vi "run.vi"(8 "error in (no error)":errorcluster, 11 "ScanModeMG090624Camera in":refnum<class "ImagingModeMG090624Camera.lvclass">) -> (0 "error out":errorcluster, 3 "ScanModeMG090624Camera out":refnum<class "ImagingModeMG090624Camera.lvclass">)   [LabVIEW 2010, in "ImagingModeMG090624Camera.lvclass"]
uses:
  ImagingModeMG090624Camera.lvclass
  common/xcontrols/XSettings/XSettings/XSettings.xctl
  common/classes/GenericComponent/GenericComponent/GenericComponent.lvclass
  main/labview_source/controls/undock_button.ctl
  ImagingModeMG090624Camera.lvclass/ImagingModeMG090624Camera.ctl
  ImagingModeDL091001Scaffold/ImagingModeDL091001Scaffold/ImagingModeDL091001Scaffold.lvclass
  ImagingModeDL091001Scaffold/ImagingModeDL091001Scaffold/internal_triggers_enum.ctl
  GenericImagingMode/GenericImagingMode/GenericImagingMode.lvclass
panel:
  in  "button:undock":T1
  in  "Tab Control":enum32{"User", "Debug", "About"}(tab)
  in  "frame rate":dbl[unit]=5.0
  in  "y resolution":i32=512
  in  "x resolution":i32=512 min=1
  in  "duration":dbl[unit]
  in  "number of frames":i32
  in  "current frame":i32
  in  "XSettings":refnum<class "GenericComponent.lvclass">(xcontrol)
  out "terminated?":bool
  out "event loop error":errorcluster
  out "XImage is user-defined?":bool
  # "frame settings"
  # "movie settings"
  # "current values"
  # "ImagingModeMG090624Camera\n\nImplemented by:\nMaurice Göldi and Dominik Langer, University of Zürich, Switzerland"
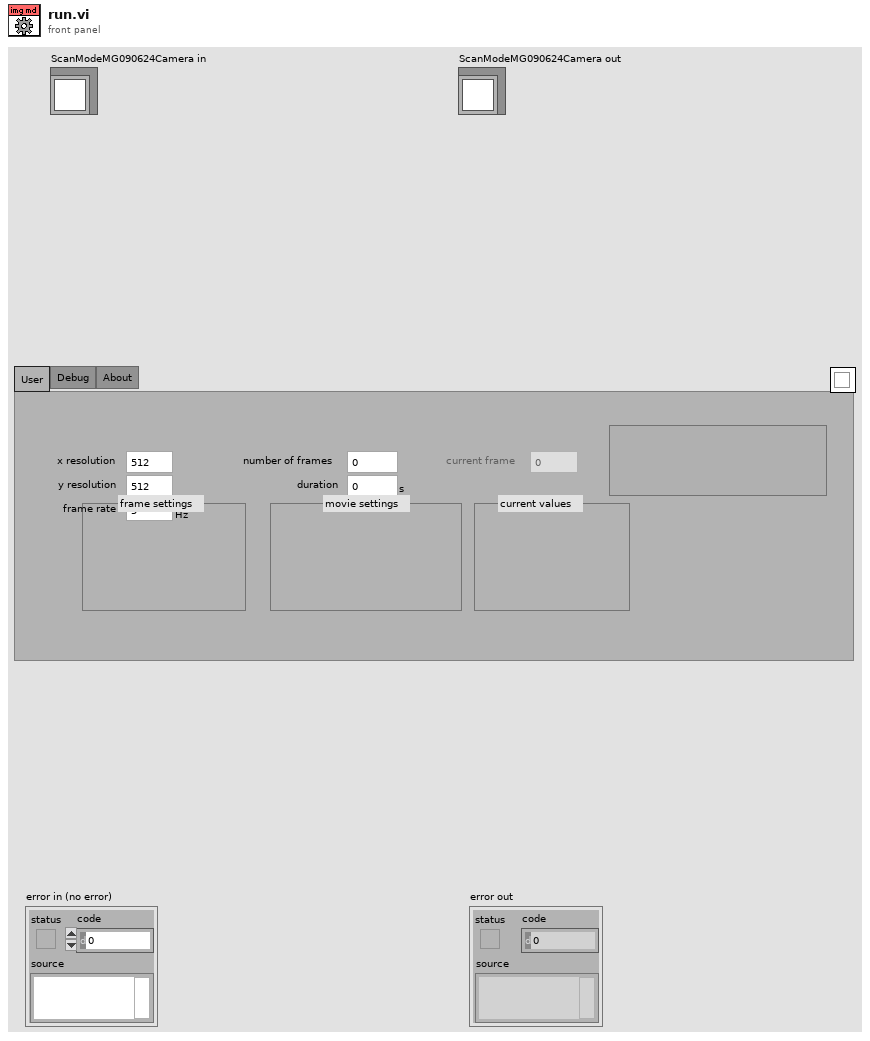
[diagram p1: front panel]
types:
  T1 = typedef "undock_button.ctl" = bool
  T2 = typedef "ImagingModeDL091001Scaffold.lvclass/internal_triggers_enum.ctl" = enum16{"NULL", "initialise", "terminate", "start sweep", "stop sweep", "update", "proceed", "draw overlay", "attach observer", "detach observer", "finish sweep"}
  T3 = enum8{"Enabled", "Disabled", "Disabled and Grayed Out"}
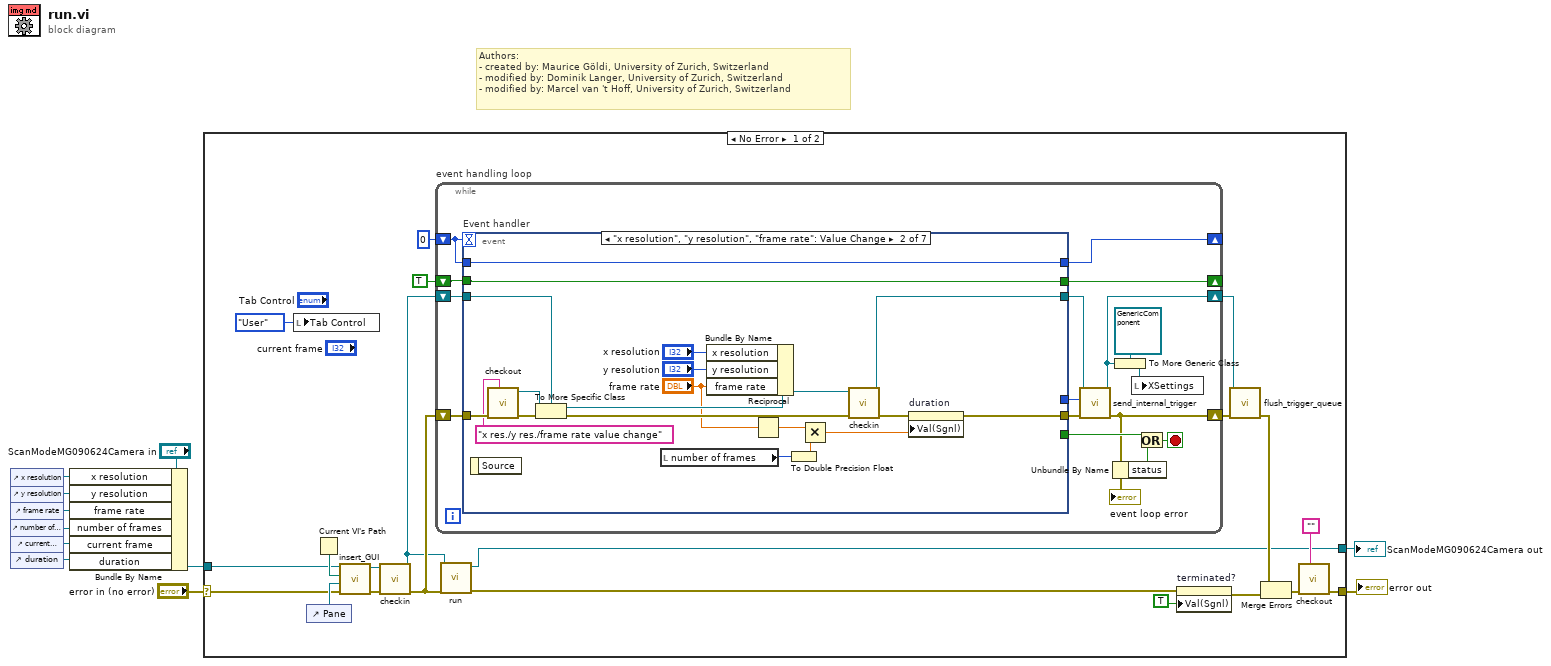
[diagram p0: block diagram]
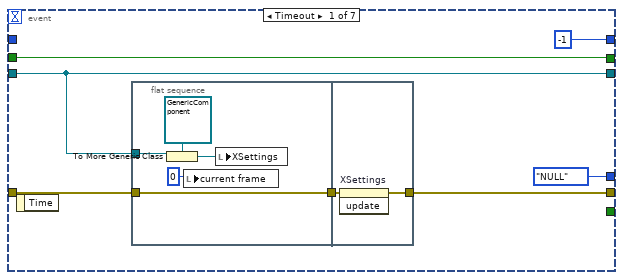
[diagram p2: hidden frame]
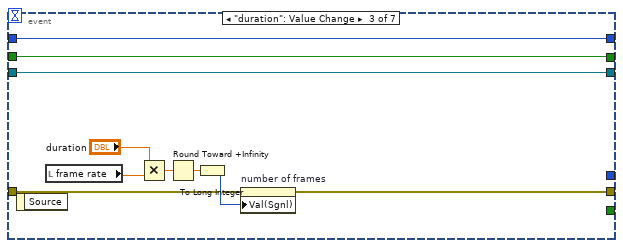
[diagram p3: hidden frame]
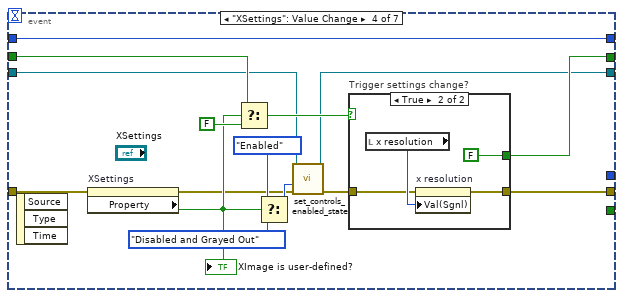
[diagram p4: hidden frame]
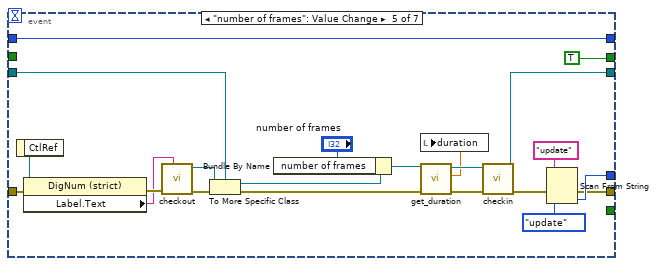
[diagram p6: hidden frame]
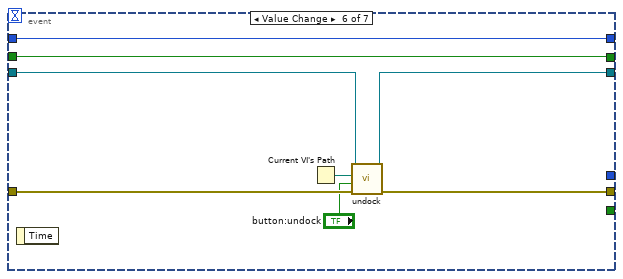
[diagram p7: hidden frame]
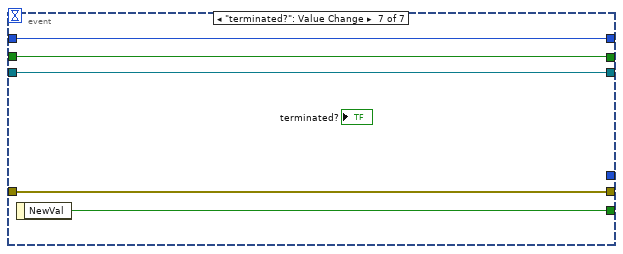
[diagram p8: hidden frame]
diagram:
  # "Authors: \n- created by: Maurice Göldi, University of Zurich, Switzerland\n- modified by: Dominik Langer, University of Zurich, Switzerland\n- modified by: Marcel van 't Hoff, University of Zurich, Switzerland"
  n1 = control-ref of="x resolution"() -> (w3:refnum<vi>)
  n2 = control-ref of="y resolution"() -> (w4:refnum<vi>)
  n3 = control-ref of="frame rate"() -> (w5:refnum<vi>)
  n4 = control-ref of="number of frames"() -> (w6:refnum<vi>)
  n5 = control-ref of="current frame"() -> (w7:refnum<vi>)
  n6 = control-ref of="duration"() -> (w8:refnum<vi>)
  n7 = Bundle By Name(cluster="ScanModeMG090624Camera in", "x resolution"=w3, "y resolution"=w4, "frame rate"=w5, "number of frames"=w6, "current frame"=w7, "duration"=w8) -> (w2:refnum<class "ImagingModeMG090624Camera.lvclass">)
  n8 = case shown="No Error" "error in (no error)" {
    selector: "error in (no error)" -> [w21 w149]
    tunnel: [w29 w149] -> w10
    tunnel: [w12 w148] -> w9
    tunnel: w2 -> [w22 w148]
    frame No Error {
      n9 = local write "Tab Control"(enum32{"User", "Debug", "About"}."User" ("Tab Control")) -> ()
      n10 = control-ref of="Pane"() -> (w23:refnum<vi>)
      n11 = Current VI's Path() -> (path=w24:path)
      n12 = call-dynamic "insert_GUI.vi"("error in (no error)"=w21, "Pane"=w23, "VI path"=w24, "GenericComponent in"=w22) -> ("error out"=w18:errorcluster, "GenericComponent out"=w17:refnum<class "ImagingModeMG090624Camera.lvclass">)  [unwired: 6 in]
      n13 = call-dynamic "checkin.vi"("error in (no error)"=w18, "GenericScanMode in"=w17) -> ("error out"=w27:errorcluster, "GenericScanMode out"=w14:refnum<class "ImagingModeMG090624Camera.lvclass">)  [unwired: 8 in]
      n14 = while "event handling loop" {
        shift-right: [w33] -> w16
        shift-left: w27 -> [w48]
        shift-right: [w46] -> _
        shift-left: 0 -> [w47]
        shift-right: [w40] -> _
        shift-left: TRUE -> [w41]
        shift-right: [w34] -> w13
        shift-left: w14 -> [w45]
        stop <- w42 stop-if-true
        n15 = event "Event handler" shown="[1] \"x resolution\", \"y resolution\", \"frame rate\": Value Change" {
          selector: _ -> [_ _ _ _ _ _ _]
          dyn-events: _ -> [_ _ _ _ _ _ _]
          timeout: w47 -> [_ _ _ _ _ _ _]
          tunnel: w48 -> [w52 w80 w86 w96 w120 w140 w147]
          tunnel: [w51 w77 w88 w99 w114 w139 w147] -> w39
          tunnel: w47 -> [_ w82 w92 w107 w134 w142 w146]
          tunnel: [-1 w82 w92 w107 w134 w142 w146] -> w46
          tunnel: w45 -> [w49 w64 w83 w94 w123 w138 w143]
          tunnel: [_ _ _ _ _ _ w145] -> w44
          tunnel: [internal_triggers_enum."NULL" ("trigger") _ _ _ w116 _ _] -> w37
          tunnel: w41 -> [w54 w72 w84 w98 _ w141 w144]
          tunnel: [w54 w72 w84 w100 TRUE w141 w144] -> w40
          tunnel: [w49 w63 w83 w93 w122 w137 w143] -> w38
          event Timeout {
            n16 = event-data() -> ()  [unwired: 2 out]
            n17 = flat-sequence {
              tunnel: w52 -> [w60]
              tunnel: [w60] -> w50
              tunnel: w49 -> [w56]
              tunnel: [w61] -> w51
              tunnel: w50 -> [w62]
              frame #0 {
                n18 = To More Generic Class(target class=refnum<class "GenericComponent.lvclass"> refnum ("GenericComponent.lvclass"), reference=w56) -> (generic class reference=w58:refnum<class "GenericComponent.lvclass">)
                n19 = local write "current frame"(0) -> ()
                n20 = local write "XSettings"(w58) -> ()
              }
              frame #1 {
                n21 = invoke on="XSettings" class="XSettings (strict)" method="update"(error in=w62) -> (error out=w61:errorcluster)  [unwired: 2 in, 2 out]
              }
            }
          }
          event "x resolution", "y resolution", "frame rate": Value Change {
            n22 = event-data() -> ()  [unwired: 2 out]
            n23 = call "checkout.vi"("locked by?"="x res./y res./frame rate value change", "error in (no error)"=w80) -> ("error out"=w81:errorcluster, "GenericScanMode out"=w79:refnum<class "GenericImagingMode.lvclass">)  [unwired: 8 in]
            n24 = To More Specific Class(target class=w64, reference=w79, error in=w81) -> (specific class reference=w76:refnum<class "ImagingModeMG090624Camera.lvclass">, error out=w71:errorcluster)
            n25 = local read "number of frames"() -> (w68:i32)
            n26 = Bundle By Name(cluster=w76, "x resolution"="x resolution", "y resolution"="y resolution", "frame rate"="frame rate") -> (w70:refnum<class "ImagingModeMG090624Camera.lvclass">)
            n27 = Reciprocal(x="frame rate") -> (1/x=w66:dbl[unit])
            n28 = To Double Precision Float(number=w68) -> (double precision float=w69:dbl)
            n29 = Multiply(x=w66, y=w69) -> (x*y=w65:dbl[unit])
            n30 = call-dynamic "checkin.vi"("error in (no error)"=w71, "GenericScanMode in"=w70) -> ("error out"=w78:errorcluster, "GenericScanMode out"=w63:refnum<class "ImagingModeMG090624Camera.lvclass">)  [unwired: 8 in]
            n31 = property on="duration" class="DigNum (strict)"(error in=w78, "Val(Sgnl)"=w65) -> (error out=w77:errorcluster)  [unwired: 1 in, 1 out]
          }
          event "duration": Value Change {
            n32 = event-data() -> ()  [unwired: 2 out]
            n33 = local read "frame rate"() -> (w85:dbl[unit])
            n34 = Multiply(x="duration", y=w85) -> (x*y=w90:dbl)
            n35 = Round Toward +Infinity(x=w90) -> (ceil(x): smallest int >= x=w89:dbl)
            n36 = To Long Integer(number=w89) -> (32bit integer=w87:i32)
            n37 = property on="number of frames" class="DigNum (strict)"(error in=w86, "Val(Sgnl)"=w87) -> (error out=w88:errorcluster)  [unwired: 1 in, 1 out]
          }
          event "XSettings": Value Change {
            n38 = event-data() -> ()  [unwired: 4 out]
            n39 = property on="XSettings" class="XSettings (strict)"(error in=w96) -> (error out=w95:errorcluster, "Property"=w97:bool)  [unwired: 1 in, 1 out]
            "XImage is user-defined?" <- w97
            n40 = Select(t=w98, s=w97, f=FALSE) -> (s? t:f=w105:bool)
            n41 = Select(t=T3."Enabled" ("status"), s=w97, f=T3."Disabled and Grayed Out" ("status")) -> (s? t:f=w104:T3)
            n42 = call-dynamic "set_controls_enabled_state.vi"("error in (no error)"=w95, "status"=w104, "GenericPlugin in"=w94) -> ("error out"=w101:errorcluster, "GenericPlugin out"=w93:refnum<class "ImagingModeMG090624Camera.lvclass">)  [unwired: 7 in]
            n43 = case "Trigger settings change?" shown="True" w105 {
              tunnel: w101 -> [w108 w110]
              tunnel: [w108 w109] -> w99
              tunnel: [_ FALSE] -> w100
              frame False {
              }
              frame True {
                n44 = local read "x resolution"() -> (w111:i32)
                n45 = property on="x resolution" class="DigNum (strict)"(error in=w110, "Val(Sgnl)"=w111) -> (error out=w109:errorcluster)  [unwired: 1 in, 1 out]
              }
            }
          }
          event "number of frames": Value Change {
            n46 = event-data() -> ("CtlRef"=w121:refnum<vi>)  [unwired: 1 out]
            n47 = property class="DigNum (strict)"(reference=w121, error in=w120) -> (error out=w119:errorcluster, "Label.Text"=w118:string)  [unwired: 1 out]
            n48 = call "checkout.vi"("locked by?"=w118, "error in (no error)"=w119) -> ("error out"=w133:errorcluster, "GenericScanMode out"=w132:refnum<class "GenericImagingMode.lvclass">)  [unwired: 8 in]
            n49 = To More Specific Class(target class=w123, reference=w132, error in=w133) -> (specific class reference=w128:refnum<class "ImagingModeMG090624Camera.lvclass">, error out=w126:errorcluster)
            n50 = Bundle By Name(cluster=w128, "number of frames"="number of frames") -> (w125:refnum<class "ImagingModeMG090624Camera.lvclass">)
            n51 = call-dynamic "get_duration.vi"("error in (no error)"=w126, "ScanModeMG090624Camera in"=w125) -> ("error out"=w131:errorcluster, "duration"=w129:dbl[unit], "ScanModeMG090624Camera out"=w130:refnum<class "ImagingModeMG090624Camera.lvclass">)  [unwired: 7 in]
            n52 = local write "duration"(w129) -> ()
            n53 = call-dynamic "checkin.vi"("error in (no error)"=w131, "GenericScanMode in"=w130) -> ("error out"=w115:errorcluster, "GenericScanMode out"=w122:refnum<class "ImagingModeMG090624Camera.lvclass">)  [unwired: 8 in]
            n54 = Scan From String(input string="update", error in=w115, default 1=internal_triggers_enum."update" ("trigger")) -> (error out=w114:errorcluster, output 1=w116:T2)  [unwired: 2 in, 2 out]
          }
          event Value Change {
            n55 = event-data() -> ()  [unwired: 2 out]
            n56 = Current VI's Path() -> (path=w135:path)
            n57 = call-dynamic "undock.vi"("error in (no error)"=w140, "undock?"="button:undock", "VI path"=w135, "component in"=w138) -> ("error out"=w139:errorcluster, "component out"=w137:refnum<class "ImagingModeMG090624Camera.lvclass">)  [unwired: 6 in]
          }
          event "terminated?": Value Change {
            n58 = event-data() -> ("NewVal"=w145:bool)  [unwired: 1 out]
          }
        }
        n59 = call-dynamic "send_internal_trigger.vi"("error in"=w39, "trigger"=w37, "ScanModeDL091001Scaffold in"=w38) -> ("error out"=w33:errorcluster, "ScanModeDL091001Scaffold out"=w34:refnum<class "ImagingModeMG090624Camera.lvclass">)  [unwired: 7 in]
        "event loop error" <- w33
        n60 = Unbundle By Name(w33) -> ("status"=w43:bool)
        n61 = To More Generic Class(target class=refnum<class "GenericComponent.lvclass"> refnum ("GenericComponent.lvclass"), reference=w34) -> (generic class reference=w35:refnum<class "GenericComponent.lvclass">)
        n62 = local write "XSettings"(w35) -> ()
        n63 = Or(x=w44, y=w43) -> (x .or. y?=w42:bool)
      }
      n64 = call-parent "run.vi"("error in (no error)"=w27, "ScanModeDL091001Scaffold in"=w14) -> ("error out"=w26:errorcluster, "ScanModeDL091001Scaffold out"=w12:refnum<class "ImagingModeMG090624Camera.lvclass">)  [unwired: 8 in]
      n65 = property on="terminated?" class="Bool (strict)"(error in=w26, "Val(Sgnl)"=TRUE) -> (error out=w28:errorcluster)  [unwired: 1 in, 1 out]
      n66 = call-dynamic "flush_trigger_queue.vi"("error in (no error)"=w16, "GenericToplevelComponent in"=w13) -> ("error out"=w15:errorcluster)  [unwired: 8 in, 1 out]
      n67 = Merge Errors(w15, w28) -> (w30:errorcluster)
      n68 = call "checkout.vi"("locked by?"="", "error in (no error)"=w30) -> ("error out"=w29:errorcluster)  [unwired: 8 in, 1 out]
    }
    frame Error {
    }
  }
  "error out" <- w10
  "ScanModeMG090624Camera out" <- w9
